vi "CS_schleife_init_mischer.vi"   [LabVIEW 2019]
uses:
  Global/Global Variables/global.vi
  Global/Global Variables/Data_Display_global.vi
  Instrument_Setup.vi
types:
  T1 = typedef "5T-Cluster.ctl" = cluster{"Go to set":bool, "Go to Zero":bool, "Clamp":bool, "Go to Hold":bool, "Clamped ":bool, "Quenched 2":bool, "Rate limit 2":bool, "Magnet (T)":dbl, "Leads (T)":dbl, "Rate (T/min)":dbl, "Sweeping":bool, "Setpoint":dbl, "Set":bool, "Zero":bool, "Hold":bool, "Clamp":bool}
  T2 = typedef "5T_Control.ctl" = cluster{"Rate (T/min)":dbl, "Setpoint":dbl, "Go to set":bool, "Go to Zero":bool, "Clamp":bool, "Go to Hold":bool, "Set Rate":bool}
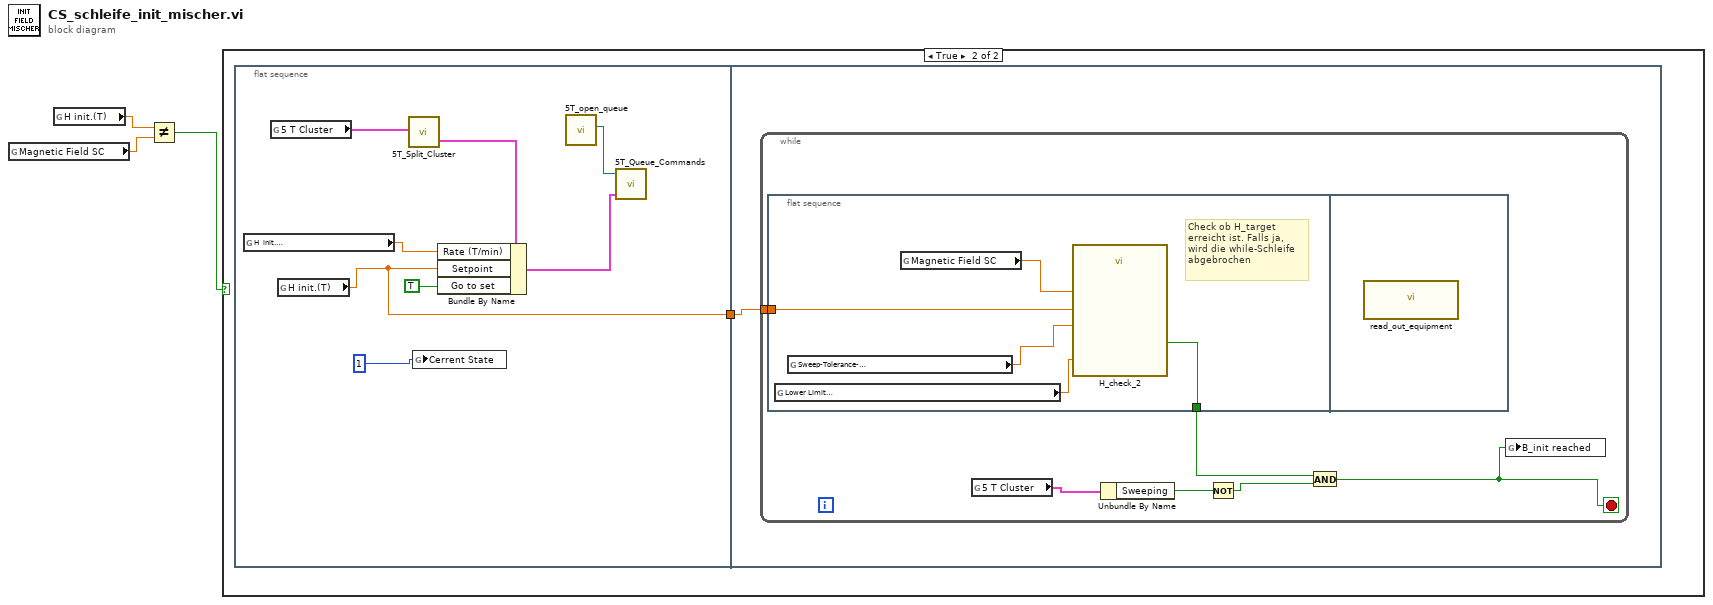
[diagram p0: block diagram]
diagram:
  n1 = global read "Data_Display_global.vi" "Magnetic Field SC"() -> (w2:dbl)
  n2 = global read "global.vi" "H init.(T)"() -> (w3:dbl)
  n3 = Not Equal?(x=w3, y=w2) -> (x != y?=w1:bool)
  n4 = case shown="True" w1 {
    frame False {
    }
    frame True {
      n5 = flat-sequence {
        tunnel: [w6] -> w4
        tunnel: w4 -> [w13]
        frame #0 {
          n6 = global read "global.vi" "H  init. \nGeschw.(T/min)"() -> (w7:dbl)
          n7 = global read "Data_Display_global.vi" "5 T Cluster"() -> (w12:T1)
          n8 = global read "global.vi" "H init.(T)"() -> (w6:dbl)
          n9 = call "5T_Split_Cluster.vi"("5 T Cluster"=w12) -> ("5T Control"=w11:T2)  [unwired: 1 out]
          n10 = global write "global.vi" "Cerrent State"(1) -> ()
          n11 = Bundle By Name(cluster=w11, "Rate (T/min)"=w7, "Setpoint"=w6, "Go to set"=TRUE) -> (w8:T2)
          n12 = call "5T_open_queue.vi"() -> ("queue out"=w9:refnum<queue>)  [unwired: 10 in, 1 out]
          n13 = call "5T_Queue_Commands.vi"("5T Control"=w8, "5T Queue"=w9) -> ()  [unwired: 1 in, 1 out]
        }
        frame #1 {
          n14 = while {
            tunnel: w13 -> [w14]
            stop <- w15 stop-if-true
            n15 = flat-sequence {
              tunnel: [w24] -> w16
              tunnel: w14 -> [w23]
              frame #0 {
                # "Check ob H_target\nerreicht ist. Falls ja,\nwird die while-Schleife\nabgebrochen"
                n16 = global read "Instrument_Setup.vi" "Lower Limit\nSweep-Tolerance-\nMagnetic-Field (T)"() -> (w20:dbl)
                n17 = global read "Instrument_Setup.vi" "Sweep-Tolerance-\nMagnetic-Field (%)"() -> (w21:dbl)
                n18 = global read "Data_Display_global.vi" "Magnetic Field SC"() -> (w22:dbl)
                n19 = call "H_check_2.vi"("Lower Limit\nSweep\nTolerance (T)"=w20, "Sweep\nTolerance %"=w21, "H_in"=w22, "H_target (K)"=w23) -> ("= H target"=w24:bool)  [unwired: 7 in]
              }
              frame #1 {
                n20 = call "read_out_equipment.vi"() -> ()  [unwired: 1 in]
              }
            }
            n21 = global read "Data_Display_global.vi" "5 T Cluster"() -> (w17:T1)
            n22 = Unbundle By Name(w17) -> ("Sweeping"=w18:bool)
            n23 = Not(x=w18) -> (.not. x?=w19:bool)
            n24 = And(x=w16, y=w19) -> (x .and. y?=w15:bool)
            n25 = global write "Data_Display_global.vi" "B_init reached"(w15) -> ()
          }
        }
      }
    }
  }
